vi "GetNumReg.vi"(10 "Ftp":refnum<k24>, 11 "error in":errorcluster) -> (2 "NumReg":dbl[](array[numeric]), 3 "error out":errorcluster)   [LabVIEW 2012, in "UnderAutomation.Fanuc.lvlib"]
uses:
  UnderAutomation.Fanuc.lvlib
  C:/Users/fg/Documents/Fanuc.vi/LabVIEW_2024/UnderAutomation.Fanuc/lib/UnderAutomation.Fanuc.dll
  LabVIEW_2024/UnderAutomation.Fanuc/lib/UnderAutomation.Fanuc.dll
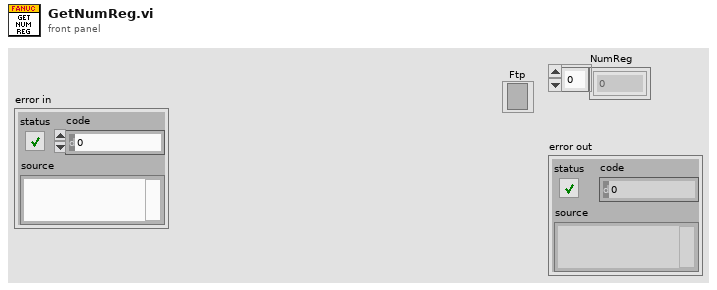
[diagram p1: front panel]
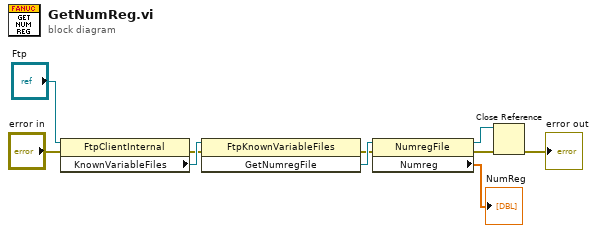
[diagram p0: block diagram]
diagram:
  n1 = property class="FtpClientInternal"(reference="Ftp", error in="error in") -> (error out=w8:errorcluster, "KnownVariableFiles"=w9:refnum<k24>)  [unwired: 1 out]
  n2 = invoke class="FtpKnownVariableFiles" method="GetNumregFile"(reference=w9, error in=w8) -> (error out=w4:errorcluster, "GetNumregFile"=w6:refnum<k24>)  [unwired: 1 in, 1 out]
  n3 = property class="NumregFile"(reference=w6, error in=w4) -> (reference out=w1:refnum<k24>, error out=w3:errorcluster, "Numreg"=→"NumReg":dbl[])
  n4 = Close Reference(reference=w1, error in (no error)=w3) -> (error out=→"error out":errorcluster)
